vi "BRig_Host_dataRunState_dataTS_dataPlot_col.vi"() -> (2 "output_idx_dataTS_dataPlot_col":i32)   [LabVIEW 2014]
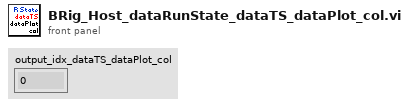
[diagram p1: front panel]
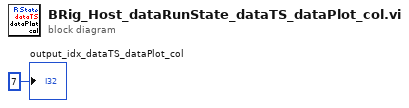
[diagram p0: block diagram]
diagram:
  "output_idx_dataTS_dataPlot_col" <- 7 ("output_idx_dataTS")
